vi "sn to n.vi"(1 "in":string) -> (0 "out":string)   [LabVIEW 2017, in "Error File Management.lvlib"]
uses:
  Error File Management.lvlib
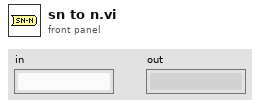
[diagram p1: front panel]
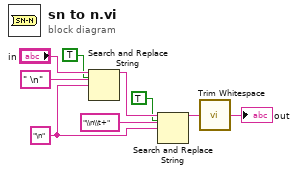
[diagram p0: block diagram]
diagram:
  w2 = "\n" ("search string")
  n1 = Search and Replace String(replace all?=TRUE ("replace all? (F)"), input string="in", search string=" \n", replace string=w2) -> (result string=w5:string)  [unwired: 4 in, 3 out]
  n2 = Search and Replace String(replace all?=TRUE ("replace all? (F)"), input string=w5, search string="\\n\\t+", replace string=w2) -> (result string=w3:string)  [unwired: 4 in, 3 out]
  n3 = call <vilib>:"Trim Whitespace.vi"("string"=w3) -> ("trimmed string"=→"out":string)  [unwired: 1 in]
